vi " Логические действия.vi"(2 "Fun":T4, 3 "B":T2, 4 "A":T3) -> (0 "Cluster":T1, 1 "Plus/min":bool)   [LabVIEW 2017]
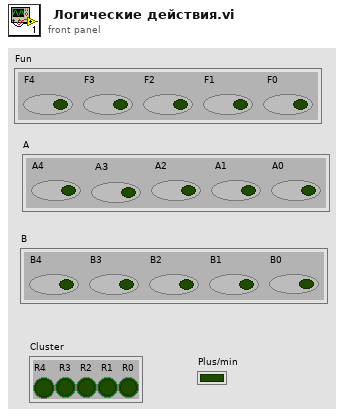
[diagram p1: front panel]
types:
  T1 = cluster{"R4":bool, " R3":bool, " R2":bool, " R1":bool, " R0":bool}
  T2 = cluster{"B4":bool, "B3":bool, "B2":bool, "B1":bool, "B0":bool}
  T3 = cluster{"A4":bool, " A3":bool, " A2":bool, " A1":bool, "A0":bool}
  T4 = cluster{"F4":bool, "F3":bool, "F2":bool, "F1":bool, " F0":bool}
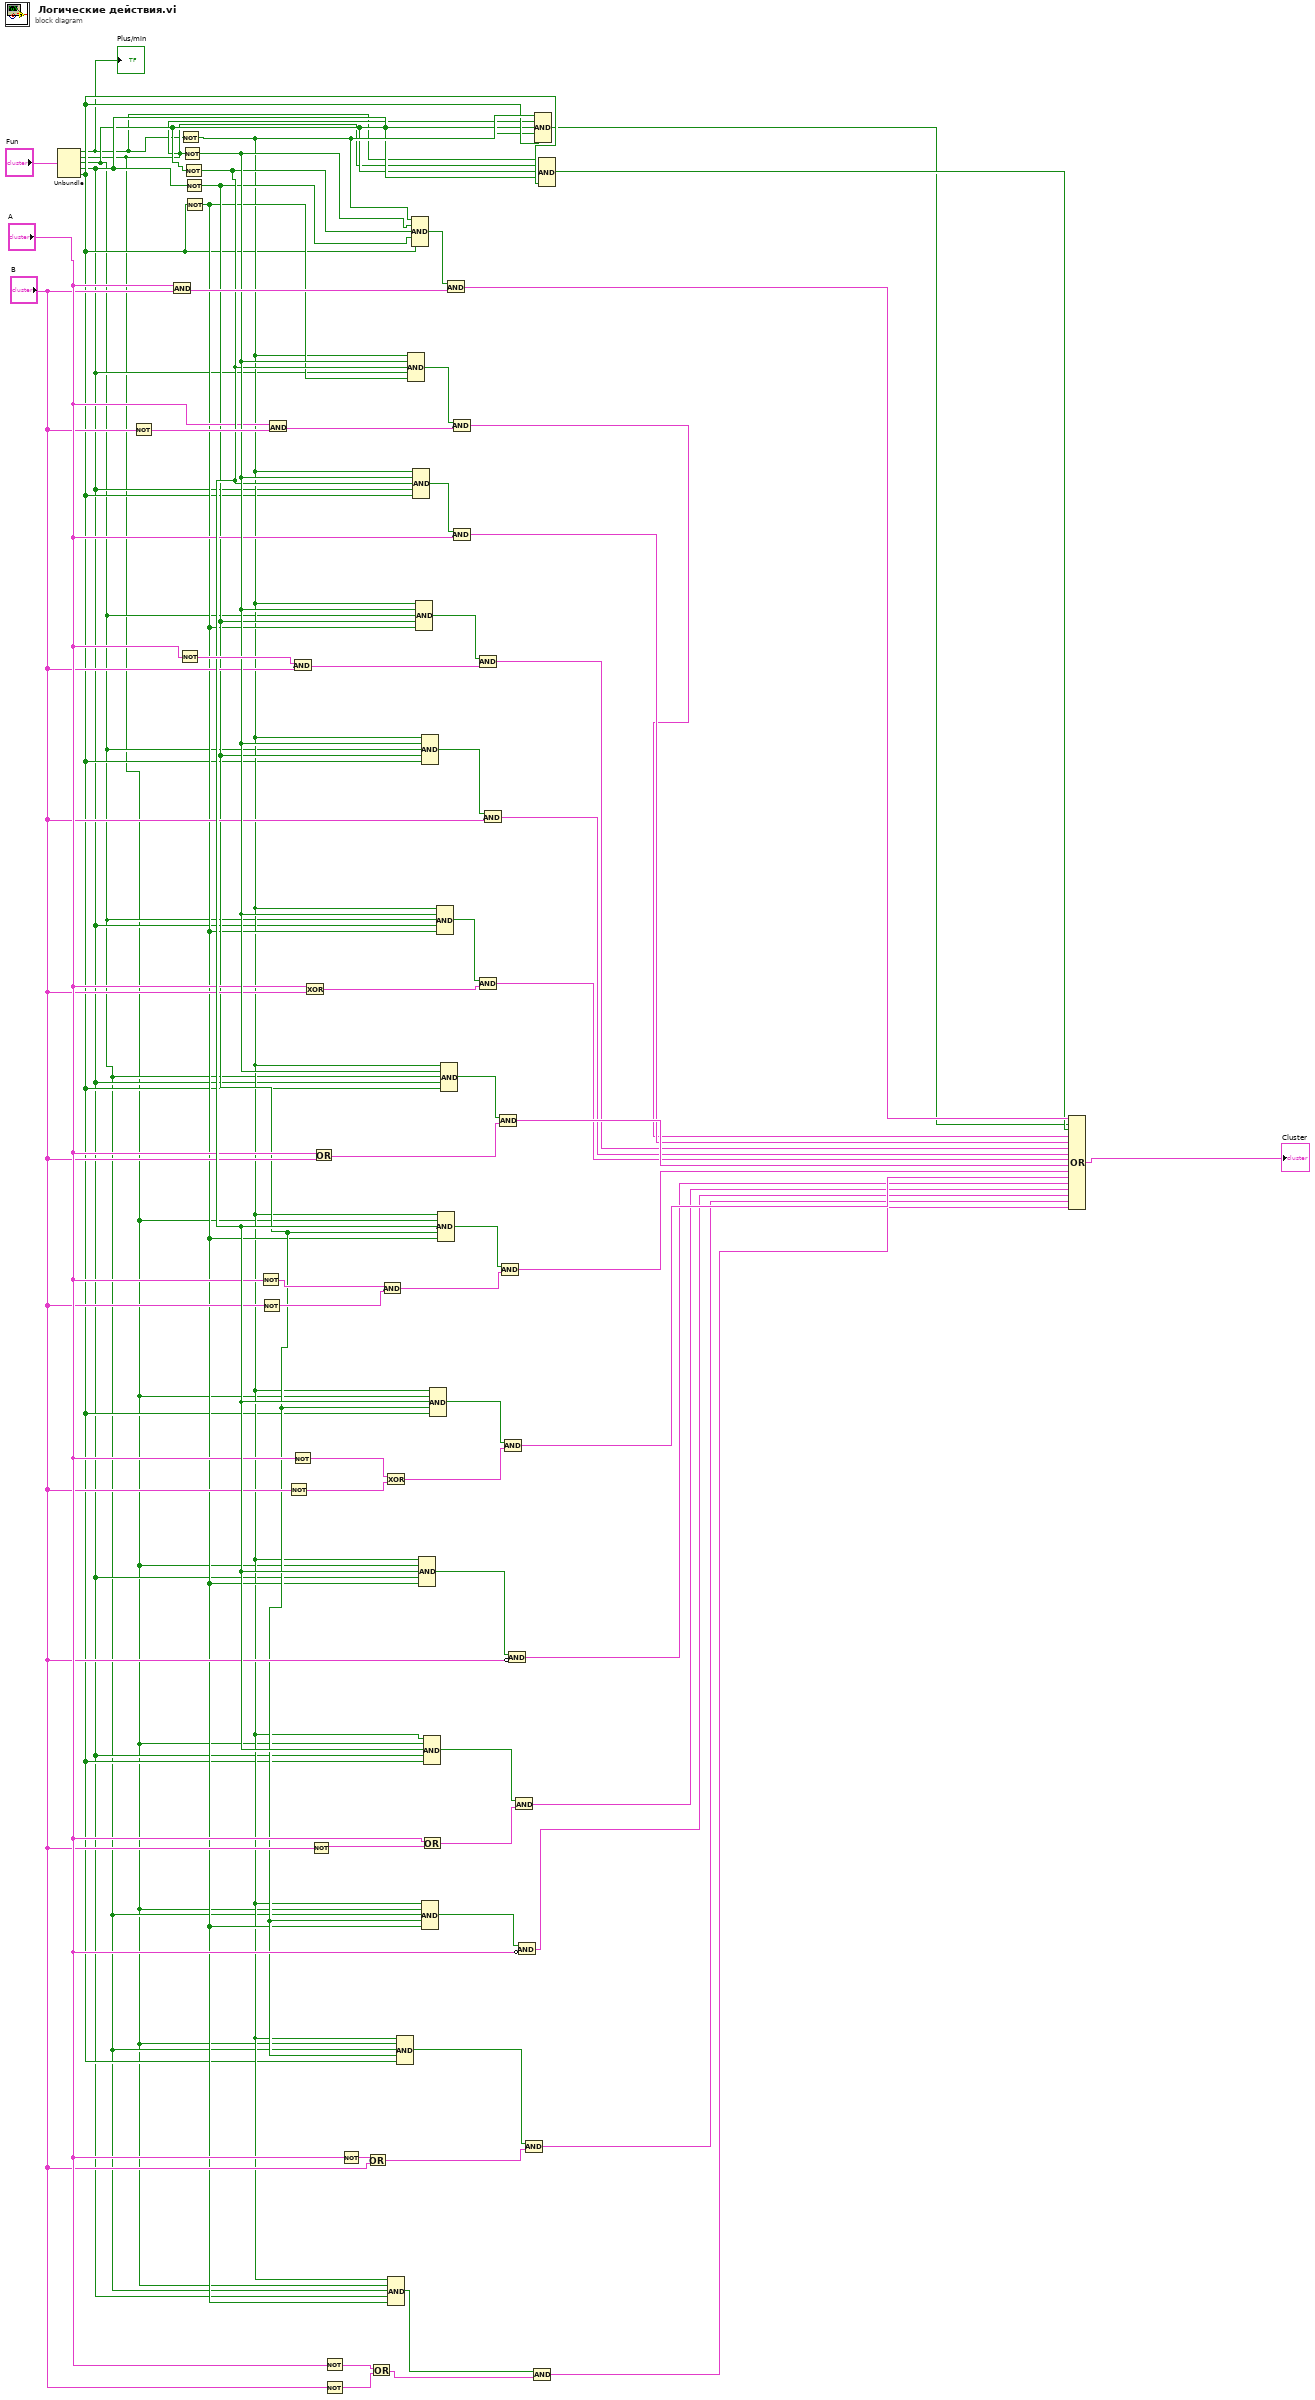
[diagram p0: block diagram]
diagram:
  n1 = Unbundle("Fun") -> ("F4"=w1:bool, "F3"=w5:bool, "F2"=w6:bool, "F1"=w7:bool, "F0"=w8:bool)
  "Plus/min" <- w1
  n2 = Not(x="B") -> (.not. x?=w62:T2)
  n3 = And(x="A", y="B") -> (x .and. y?=w63:cluster{bool, bool, bool, bool, bool})
  n4 = Not(x="A") -> (.not. x?=w57:T3)
  n5 = Not(x=w1) -> (.not. x?=w9:bool)
  n6 = Not(x=w5) -> (.not. x?=w31:bool)
  n7 = Not(x=w6) -> (.not. x?=w27:bool)
  n8 = Not(x=w7) -> (.not. x?=w13:bool)
  n9 = Not(x=w8) -> (.not. x?=w12:bool)
  n10 = Not(x="A") -> (.not. x?=w40:T3)
  n11 = Not(x="B") -> (.not. x?=w39:T2)
  n12 = And(x="A", y=w62) -> (x .and. y?=w61:cluster{bool, bool, bool, bool, bool})
  n13 = Not(x="B") -> (.not. x?=w38:T2)
  n14 = And(x=w57, y="B") -> (x .and. y?=w56:cluster{bool, bool, bool, bool, bool})
  n15 = Not(x="A") -> (.not. x?=w37:T3)
  n16 = Exclusive Or(1:"B", 2:"A") -> (0:w52:cluster{bool, bool, bool, bool, bool})
  n17 = Not(x="B") -> (.not. x?=w30:T2)
  n18 = Or(x="A", y="B") -> (x .or. y?=w50:cluster{bool, bool, bool, bool, bool})
  n19 = Not(x="A") -> (.not. x?=w20:T3)
  n20 = Not(x="B") -> (.not. x?=w19:T2)
  n21 = Not(x="A") -> (.not. x?=w22:T3)
  n22 = Or(x=w22, y="B") -> (x .or. y?=w21:cluster{bool, bool, bool, bool, bool})
  n23 = Or(x=w20, y=w19) -> (x .or. y?=w16:cluster{bool, bool, bool, bool, bool})
  n24 = And(x=w40, y=w39) -> (x .and. y?=w41:cluster{bool, bool, bool, bool, bool})
  n25 = Exclusive Or(1:w38, 2:w37) -> (0:w35:cluster{bool, bool, bool, bool, bool})
  n26 = Compound Arithmetic op=AND(w9, w5, w6, w7, w12) -> (w15:bool)
  n27 = Compound Arithmetic op=AND(w9, w5, w6, w13, w8) -> (w14:bool)
  n28 = Compound Arithmetic op=AND(w9, w31, w27, w7, w12) -> (w58:bool)
  n29 = Compound Arithmetic op=AND(w9, w31, w27, w13, w8) -> (w60:bool)
  n30 = Compound Arithmetic op=AND(w9, w31, w27, w7, w8) -> (w59:bool)
  n31 = Compound Arithmetic op=AND(w9, w31, w6, w13, w12) -> (w55:bool)
  n32 = Compound Arithmetic op=AND(w9, w5, w27, w7, w12) -> (w32:bool)
  n33 = Or(x="A", y=w30) -> (x .or. y?=w28:cluster{bool, bool, bool, bool, bool})
  n34 = Compound Arithmetic op=AND(w9, w31, w6, w13, w8) -> (w54:bool)
  n35 = Compound Arithmetic op=AND(w9, w5, w6, w13, w12) -> (w24:bool)
  n36 = Compound Arithmetic op=AND(w9, w5, w27, w7, w8) -> (w29:bool)
  n37 = Compound Arithmetic op=AND(w9, w5, w27, w13, w8) -> (w36:bool)
  n38 = Compound Arithmetic op=AND(w9, w31, w6, w7, w12) -> (w53:bool)
  n39 = Compound Arithmetic op=AND(w9, w5, w27, w13, w12) -> (w49:bool)
  n40 = Compound Arithmetic op=AND(w9, w31, w6, w7, w8) -> (w51:bool)
  n41 = Compound Arithmetic op=AND(w60, w63) -> (w33:cluster{bool, bool, bool, bool, bool})
  n42 = Compound Arithmetic op=AND(w58, w61) -> (w42:cluster{bool, bool, bool, bool, bool})
  n43 = Compound Arithmetic op=AND(w59, "A") -> (w43:T3)
  n44 = Compound Arithmetic op=AND(w53, w52) -> (w46:cluster{bool, bool, bool, bool, bool})
  n45 = Compound Arithmetic op=AND(w55, w56) -> (w44:cluster{bool, bool, bool, bool, bool})
  n46 = Compound Arithmetic op=AND(w54, "B") -> (w45:T2)
  n47 = Compound Arithmetic op=AND(w51, w50) -> (w47:cluster{bool, bool, bool, bool, bool})
  n48 = Compound Arithmetic op=AND(w49, w41) -> (w48:cluster{bool, bool, bool, bool, bool})
  n49 = Compound Arithmetic op=AND(w36, w35) -> (w34:cluster{bool, bool, bool, bool, bool})
  n50 = Compound Arithmetic op=AND(w32, invert "B") -> (w26:T2)
  n51 = Compound Arithmetic op=AND(w29, w28) -> (w25:cluster{bool, bool, bool, bool, bool})
  n52 = Compound Arithmetic op=AND(w24, invert "A") -> (w23:T3)
  n53 = Compound Arithmetic op=AND(w14, w21) -> (w11:cluster{bool, bool, bool, bool, bool})
  n54 = Compound Arithmetic op=AND(w15, w16) -> (w10:cluster{bool, bool, bool, bool, bool})
  n55 = Compound Arithmetic op=AND(w9, w5, w6, w7, w8) -> (w2:bool)
  n56 = Compound Arithmetic op=AND(w1, w5, w6, w7, w8) -> (w3:bool)
  n57 = Compound Arithmetic op=OR(w33, w2, w3, w42, w43, w44, w45, w46, w47, w48, w34, w26, w25, w23, w11, w10) -> (→"Cluster":cluster{bool, bool, bool, bool, bool})
